vi "Get GUI Item Value - Integer.vi"(7 "Default":i32, 8 "error in (no error)":errorcluster, 10 "FP Item Name":string, 11 "uService Template in":refnum<class "Father of all uServices.lvclass">) -> (0 "error out":errorcluster, 2 "Value":i32, 3 "uService Template out":refnum<class "Father of all uServices.lvclass">)   [LabVIEW 2026, in "TALOS.lvlib" / "Father of all uServices.lvlib" / "Father of all uServices.lvclass"]
doc: "Returns the value currently present in the µService GUI Indicator (or control - to be verified) with the name (label) provided. Brother methods are created to already provide the correct datatype in output (Bool, Str, Dbl, Int)."
uses:
  Father of all uServices.lvclass
  Ancestor/Ancestor/Ancestor.lvclass/Ancestor.ctl
  Support VIs/Generate Error.vi
  FGV/Error Memory/Get Error Description.vi
  Support VIs/Get PC name.vi
  Ancestor/Ancestor/Read ID.vi
  Support VIs/Get Class Name.vi
  <vilib>/Utility/error.llb/Clear Errors.vi
  FGV/Error Memory/Error Memory Core.vi
  <vilib>/AdvancedString/Delimited String to 1D String Array.vi
  <vilib>/AdvancedString/Delimited String to 1D String Array (string).vi
  Support VIs/Circus Root Path.vi
  FGV/Error Memory/Error Crt Lvl checker.vi
  FGV/Error Memory/Error Memory Core.vi/40c8088d-b597-4017-91af-faa98e00292e.vi
  FGV/Error Memory/Error Memory Core.vi/d4a3ab98-063c-4e44-b43d-fbdcfe6c2be2.vi
  Support VIs/Global Memory.vi
  <vilib>/Utility/LVClass/Get LV Class Name.vi
  Support VIs/Is in Packed Library.vi
  Support VIs/TALOS Root path.vi
  Support VIs/Read CSV worksheet.vi
  Support VIs/Global Constants.vi
  <vilib>/Utility/error.llb/General Error Handler.vi
  Support VIs/Error Log.vi
  Ancestor/Ancestor/Ancestor.lvclass
  <vilib>/Comparison/Equal/Equal Functor/Equal Functor.lvclass
  TALOS.lvlib
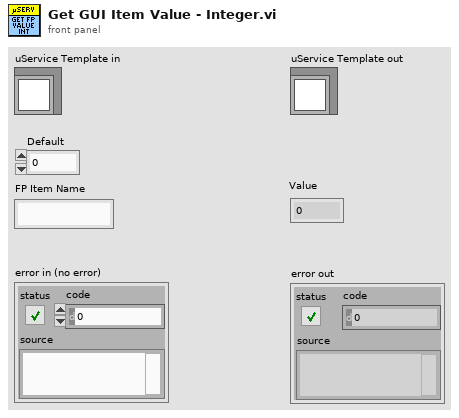
[diagram p1: front panel]
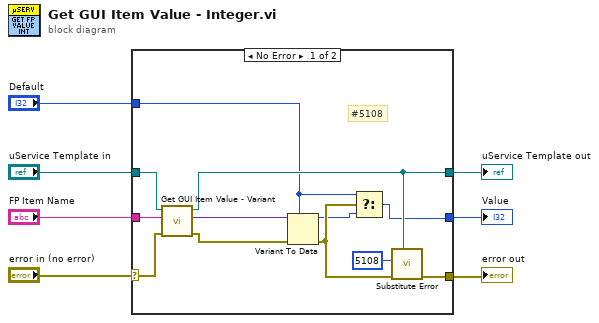
[diagram p0: block diagram]
diagram:
  n1 = case shown="No Error" "error in (no error)" {
    selector: "error in (no error)" -> [w16 w22]
    tunnel: [w19 w21] -> w7
    tunnel: [w9 w20] -> w6
    tunnel: "FP Item Name" -> [w15 _]
    tunnel: "uService Template in" -> [w14 w21]
    tunnel: [w13 w22] -> w2
    tunnel: "Default" -> [w8 w20]
    frame No Error {
      # "#5108"
      n2 = call "Get GUI Item Value - Variant.vi"("error in (no error)"=w16, "FP Item Name"=w15, "uService Template in"=w14) -> ("error out"=w17:errorcluster, "Value"=w18:variant, "uService Template out"=w19:refnum<class "Father of all uServices.lvclass">)  [unwired: 6 in]
      n3 = Variant To Data(error in=w17, type=w8, Variant=w18) -> (data=w10:i32, error out=w11:errorcluster)
      n4 = Select(t=w8, s=w11, f=w10) -> (s? t:f=w9:i32)
      n5 = call "Substitute Error.vi"("LabVIEW Object"=w19, "error in (no error)"=w11, "Error Code"=5108) -> ("error out"=w13:errorcluster)  [unwired: 8 in]
    }
    frame Error {
    }
  }
  "error out" <- w2
  "uService Template out" <- w7
  "Value" <- w6
